vi "Initialize Session.vi"(8 "error in (no error)":errorcluster, 9 "Initialize_Info":T1, 10 "session reservation":refnum<class "Session Reservation.lvclass">, 11 "NI-DMM in":refnum<class "niDCPower.lvclass">) -> (0 "error out":errorcluster, 3 "NI-DMM out":refnum<class "niDCPower.lvclass">)   [LabVIEW 2021, in "niDCPower.lvclass"]
uses:
  niDCPower.lvclass
  TypeDefs/Initialize_Info.ctl
  <vilib>/Plug-In SDKs/Clients/Session Management V1/Session Reservation/Initialize and Close Session Behavior.ctl
  <vilib>/Plug-In SDKs/Clients/Session Management V1/Session Reservation/Session Reservation.lvclass
  niDCPower.lvclass/niDCPower.ctl
  <vilib>/Plug-In SDKs/Sessions/niDCPower/Initialize Sessions - 1Sess.vi
  <vilib>/Plug-In SDKs/Sessions/niDCPower/NI Session Management niDCPower.lvlib
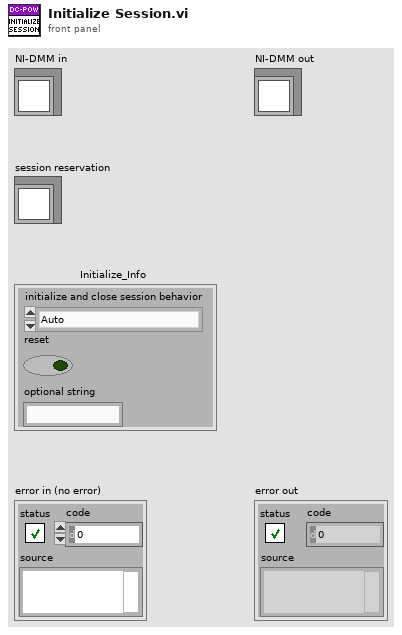
[diagram p1: front panel]
types:
  T1 = typedef "niDCPower.lvclass/Initialize_Info.ctl" = cluster{"initialize and close session behavior":T2, "reset":bool, "optional string":string}
  T2 = typedef "NI Session Management V1 Client.lvlib/Session Reservation.lvclass/Initialize and Close Session Behavior.ctl" = enum16{"Auto", "Initialize and Close", "Attach and Detach", "Initialize and Detach", "Attach and Close"}
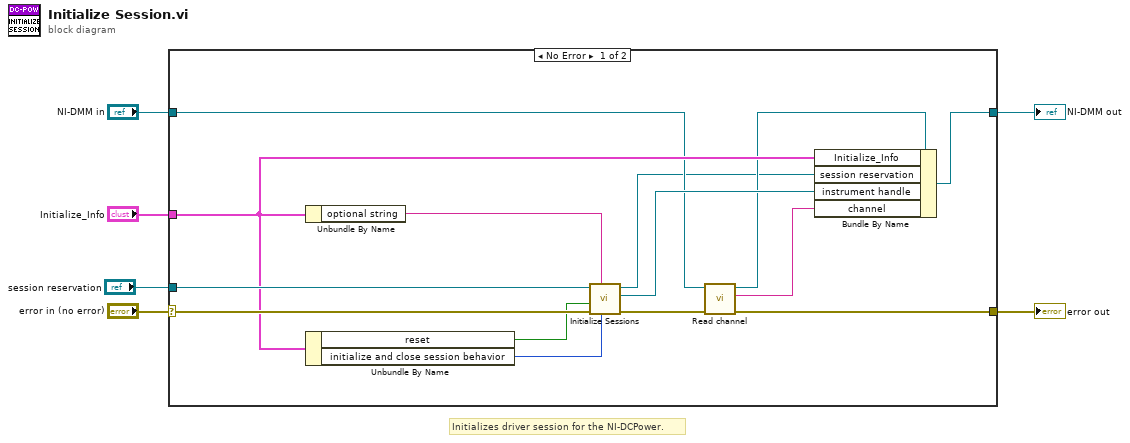
[diagram p0: block diagram]
diagram:
  # "Initializes driver session for the NI-DCPower."
  n1 = case shown="No Error" "error in (no error)" {
    selector: "error in (no error)" -> [w19 w22]
    tunnel: "NI-DMM in" -> [w9 w21]
    tunnel: [w11 w22] -> w4
    tunnel: [w20 w21] -> w3
    tunnel: "Initialize_Info" -> [w13 _]
    tunnel: "session reservation" -> [w14 _]
    frame No Error {
      n2 = Unbundle By Name(w13) -> ("optional string"=w16:string)
      n3 = Unbundle By Name(w13) -> ("reset"=w18:bool, "initialize and close session behavior"=w17:T2)
      n4 = call-poly <vilib>:"Initialize Sessions.vi"("initialize and close session behavior"=w17, "option string"=w16, "error in"=w19, "reset"=w18, "session reservation in"=w14) -> ("error out"=w12:errorcluster, "session"=w15:refnum<k15>, "session reservation out"=w7:refnum<class "Session Reservation.lvclass">)  [unwired: 3 in, 1 out]
      n5 = call-dynamic "Read channel.vi"("error in (no error)"=w12, "Abstract_Instrument in"=w9) -> ("error out"=w11:errorcluster, "channel"=w8:string, "Abstract_Instrument out"=w10:refnum<class "niDCPower.lvclass">)  [unwired: 7 in]
      n6 = Bundle By Name(cluster=w10, "Initialize_Info"=w13, "session reservation"=w7, "instrument handle"=w15, "channel"=w8) -> (w20:refnum<class "niDCPower.lvclass">)
    }
    frame Error {
    }
  }
  "error out" <- w4
  "NI-DMM out" <- w3
